vi "delete_head.vi"(8 "error in (no error)":errorcluster, 11 "DoublyLinkedList in":refnum<class "DoublyLinkedList.lvclass">) -> (0 "error out":errorcluster, 3 "DoublyLinkedList out":refnum<class "DoublyLinkedList.lvclass">)   [LabVIEW 2021, in "DoublyLinkedList.lvclass"]
uses:
  DoublyLinkedList.lvclass
  DoublyLinkedList.lvclass/DoublyLinkedList.ctl
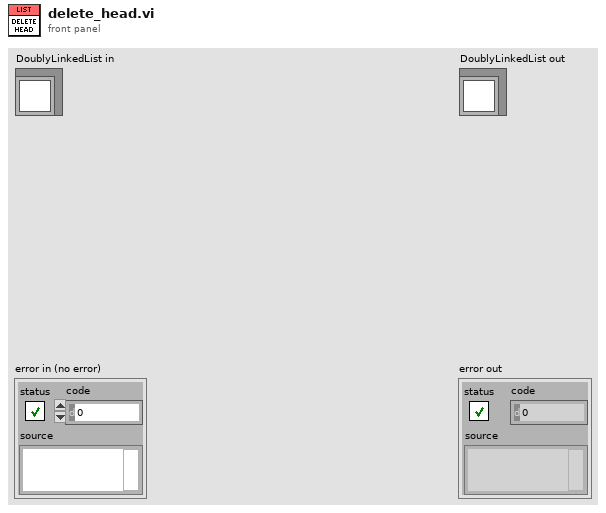
[diagram p1: front panel]
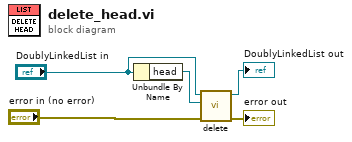
[diagram p0: block diagram]
diagram:
  n1 = Unbundle By Name("DoublyLinkedList in") -> ("head"=w5:refnum<class "DoublyNodeRef.lvclass">)
  n2 = call-dynamic "delete.vi"("error in (no error)"="error in (no error)", "current node"=w5, "DoublyLinkedList in"="DoublyLinkedList in") -> ("error out"=→"error out":errorcluster, "DoublyLinkedList out"=→"DoublyLinkedList out":refnum<class "DoublyLinkedList.lvclass">)  [unwired: 7 in]
